vi "Print_Barcode.vi"(6 "RePrint":bool, 8 "error in (no error)":errorcluster, 9 "User Data":T1, 10 "RFID":string, 11 "Ref in":T2={"MS SQL Connection"=refnum, "UDL File"=path "", "Time"="", "DCODE"="", "WIP+1"=0, "MC No?"=0, "POKAYOKE?"=FALSE, "Expected Result"="", "Result [Status]"="", "Clock"=0.0, "RFID"="", "WIP Queue"=refnum, "TS Parameter"={"ProfitCenterCode"="", "LineCode"="", "WorkOrderNumber"="", "Model"="", "Model_with_Prefix"="", "VendorCode"="", "SetParameterDateCode"="", "PokaYoke"=0, "Target"=1, "Live_DateCode"="", "CustomerPartNumber"="", "Hand"="", "sBarcode"=FALSE, "FCA"=0, "Ent_Stamp"=timestamp(0 s since 1904-01-01), "STS_CD"=0.0}, "Data_Queue"=[], "RFID Serial No."=""} {"TS Parameter"."FCA" format="%01d"; "TS Parameter"."Target" min=1 max=100000; "TS Parameter"."PokaYoke" min=0 max=1}) -> (0 "error out":errorcluster, 1 "Serial No.":i32, 2 "Barcode":string, 3 "Ref Out":T2={"MS SQL Connection"=refnum, "UDL File"=path "", "Time"="", "DCODE"="", "WIP+1"=0, "MC No?"=0, "POKAYOKE?"=FALSE, "Expected Result"="", "Result [Status]"="", "Clock"=0.0, "RFID"="", "WIP Queue"=refnum, "TS Parameter"={"ProfitCenterCode"="", "LineCode"="", "WorkOrderNumber"="", "Model"="", "Model_with_Prefix"="", "VendorCode"="", "SetParameterDateCode"="", "PokaYoke"=0, "Target"=1, "Live_DateCode"="", "CustomerPartNumber"="", "Hand"="", "sBarcode"=FALSE, "FCA"=0, "Ent_Stamp"=timestamp(0 s since 1904-01-01), "STS_CD"=0.0}, "Data_Queue"=[], "RFID Serial No."=""} {"TS Parameter"."FCA" format="%01d"; "TS Parameter"."Target" min=1 max=100000; "TS Parameter"."PokaYoke" min=0 max=1}, 4 "Last Printed BC Mirror":string, 5 "Print Time":string, 7 "resulting string":string)   [LabVIEW 2020]
uses:
  Controls/TD SQL.ctl
  <vilib>/addons/database/Connection.llb/Conn ObjectReference.ctl
  Controls/WIP_State.ctl
  Controls/TS_Parameter.ctl
  Controls/user_log.ctl
  <vilib>/addons/database/Connection.llb/Conn Execute.vi
  <vilib>/addons/database/Recordset.llb/Rec Fetch Recordset Data (R).vi
  <vilib>/addons/database/Recordset.llb/Rec Destroy - Connection.vi
  <vilib>/addons/database/_DB Variant To Data/Database Variant To Data.xnode
  <vilib>/addons/database/NI_Database_API.lvlib
panel:
  out "match substring":string
  out "Pass Date":timestamp
  out "element":string
  out "Total Seconds 2":i32
  out "substring":string
  out "text 2":string
  out "Total Seconds":i32
  out "text":string
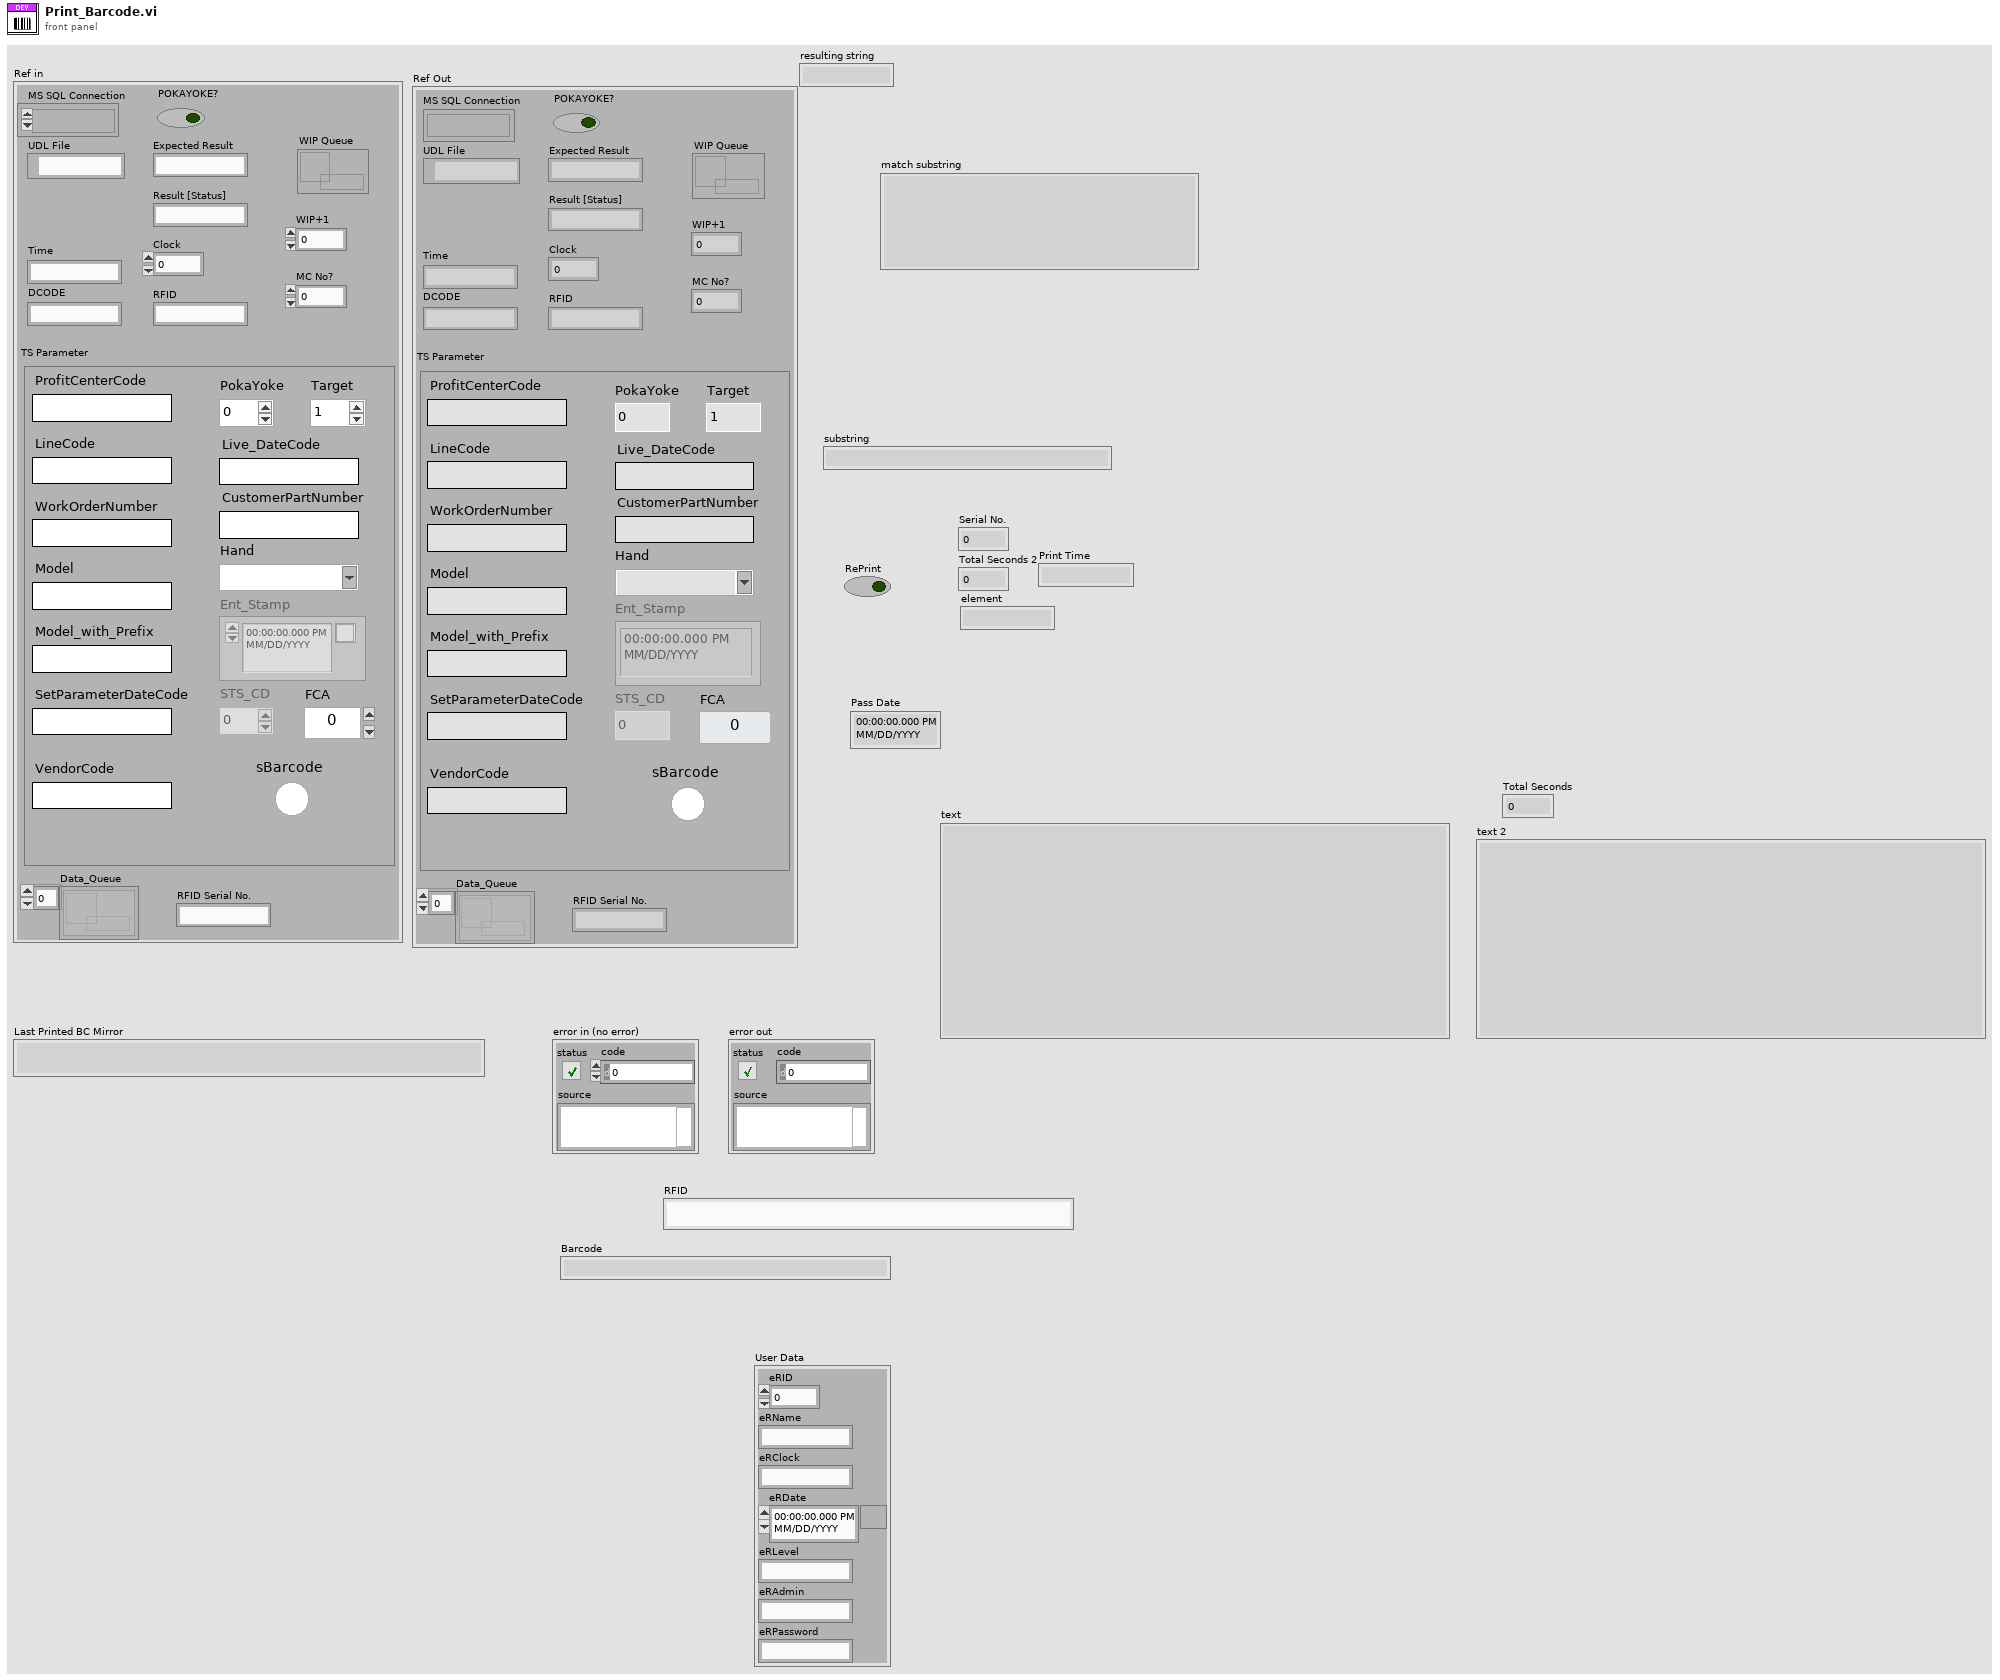
[diagram p1: front panel]
types:
  T1 = typedef "user_log.ctl" = cluster{"eRID":u16, "eRName":string, "eRClock":string, "eRDate":timestamp, "eRLevel":string, "eRAdmin":string, "eRPassword":string}
  T2 = typedef "TD SQL.ctl" = cluster{"MS SQL Connection":T3, "UDL File":path, "Time":string, "DCODE":string, "WIP+1":i64, "MC No?":i32, "POKAYOKE?":bool, "Expected Result":string, "Result [Status]":string, "Clock":dbl, "RFID":string, "WIP Queue":refnum<queue>, "TS Parameter":T4, "Data_Queue":refnum<queue>[], "RFID Serial No.":string}
  T3 = typedef "NI_Database_API.lvlib/Conn ObjectReference.ctl" = refnum<k1>
  T4 = typedef "TS_Parameter.ctl" = cluster{"ProfitCenterCode":string, "LineCode":string, "WorkOrderNumber":string, "Model":string, "Model_with_Prefix":string, "VendorCode":string, "SetParameterDateCode":string, "PokaYoke":i32, "Target":i32, "Live_DateCode":string, "CustomerPartNumber":string, "Hand":string, "sBarcode":bool, "FCA":i32, "Ent_Stamp":timestamp, "STS_CD":dbl}
  T5 = cluster{"CUSTOMER PART NUMBER":string, "Version Number":string, "VENDOR CODE":string, "BI PART NUMBER":string, "SCAN TYPE":enum16{"AUTO", "MANUAL"}, "BARCODE TYPE":enum16{"X451", "MSIL-YNC10 Trial1"}, "CELL NUMBER":string}
  T6 = enum16{"open", "replace", "create", "open or create", "replace or create", "replace or create with confirmation"}
  T7 = typedef "NI_Database_API.lvlib/Rec ObjectReference.ctl" = refnum<k1>
  T8 = cluster{"Data Path":path, "Calibration Path":path, "Settings Path":path, "Script Path":path, "DAQ Support":path, "Reporting Desktop":path, "Help":path}
  T9 = typedef "LVDateTimeRec.ctl" = cluster{"fractional second":dbl, "second":i32, "minute":i32, "hour":i32, "day of month":i32, "month":i32, "year":i32, "day of week":i32, "day of year":i32, "DST":i32}
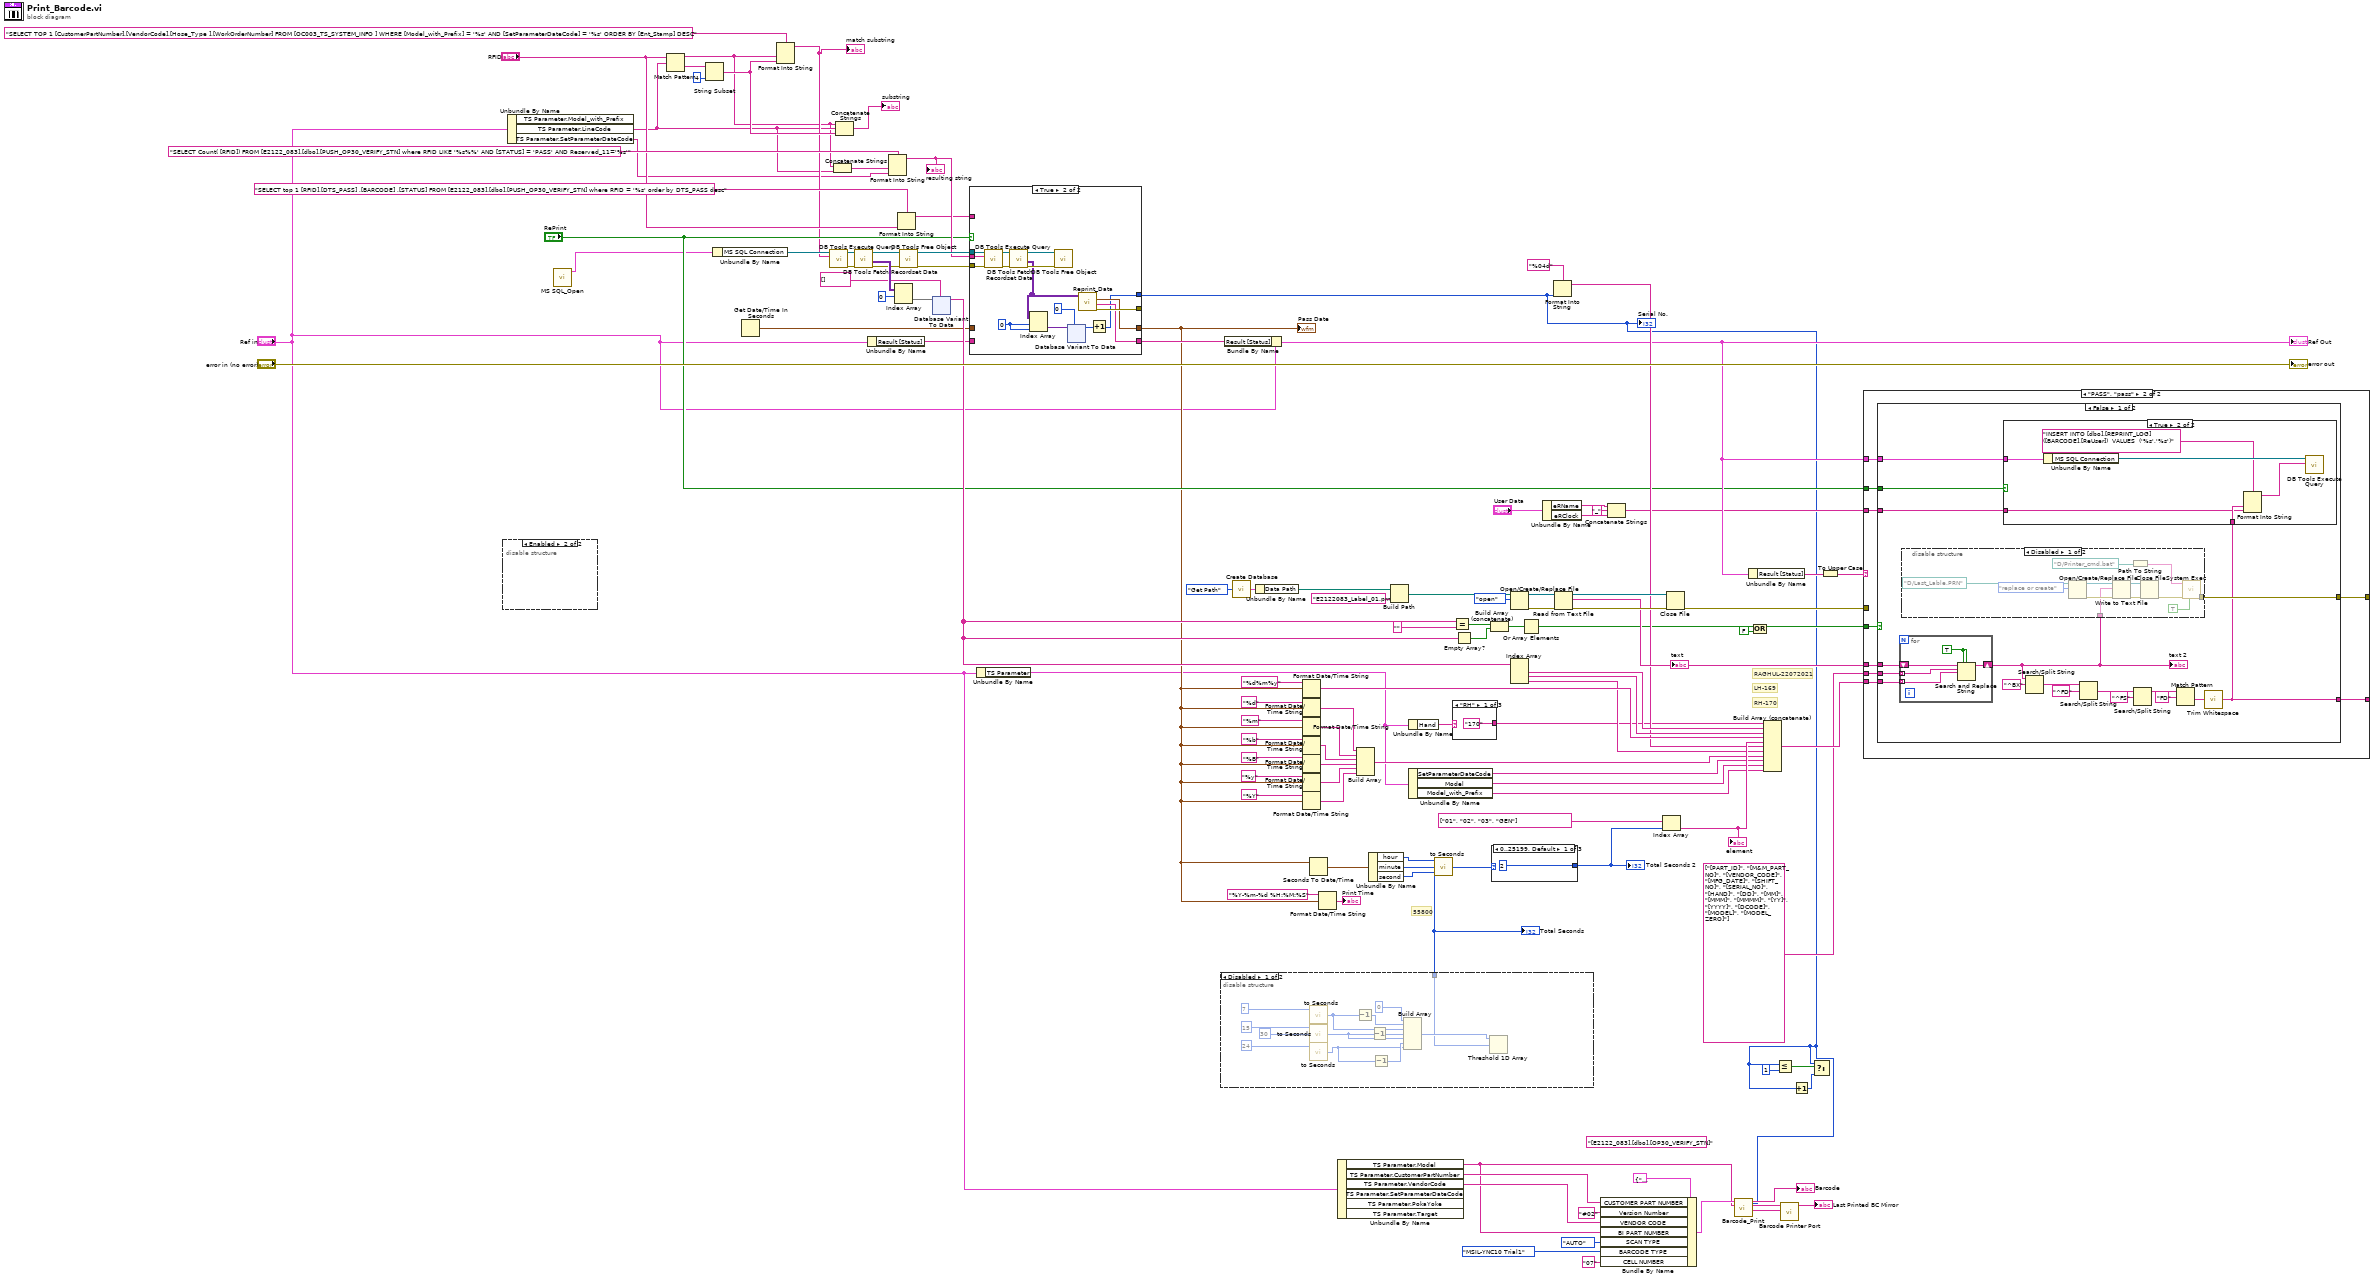
[diagram p0: block diagram]
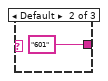
[diagram p2: hidden frame]
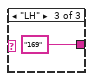
[diagram p3: hidden frame]
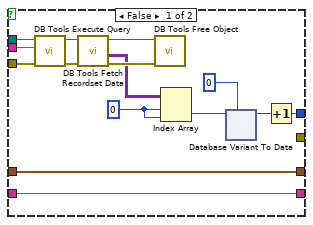
[diagram p5: hidden frame]
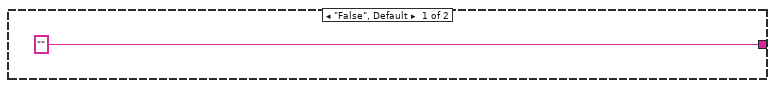
[diagram p6: hidden frame]
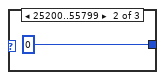
[diagram p11: hidden frame]
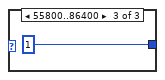
[diagram p12: hidden frame]
diagram:
  (unwired) "[E2122_083].[dbo].[OP30_VERIFY_STN]" ("table")
  # "RAGHUL-22072021"
  # "RH-170"
  # "LH-169"
  # "55800"
  n1 = disable-structure shown="Enabled" {
    frame Disabled {
    }
    frame Enabled {
    }
  }
  n2 = Unbundle By Name("Ref in") -> ("TS Parameter.LineCode"=w5:string, "TS Parameter.SetParameterDateCode"=w3:string)  [unwired: 1 out]
  n3 = call "MS SQL_Open.vi"() -> ("Ref Out"=w22:T2)  [unwired: 9 in, 2 out]
  n4 = Match Pattern(string="RFID", regular expression=w5) -> (before substring=w2:string, after substring=w76:string)  [unwired: 1 in, 2 out]
  n5 = String Subset(string=w76, length (rest)=4 ("length (rest)")) -> (substring=w59:string)  [unwired: 1 in]
  n6 = Unbundle By Name(w22) -> ("MS SQL Connection"=w68:T3)
  n7 = Get Date/Time In Seconds() -> (seconds since 1Jan1904=w35:timestamp)
  n8 = Format Into String(format string="SELECT TOP 1 [CustomerPartNumber],[VendorCode],[Hose_Type ],[WorkOrderNumber] FROM [OC003_TS_SYSTEM_INFO ] WHERE [Model_with_Prefix] = '%s' AND [SetParameterDateCode] = '%s' ORDER BY [Ent_Stamp] DESC" ("condition"), w2, w59) -> (resulting string=w23:string)  [unwired: 2 in, 1 out]
  "match substring" <- w23
  n9 = call-poly <vilib>:"DB Tools Execute Query.vi"("SQL query"=w23, "connection reference"=w68) -> ("error out"=w72:errorcluster, "recordset reference"=w73:T7)  [unwired: 6 in]
  n10 = Concatenate Strings(w2, w5) -> (w4:string)
  n11 = Concatenate Strings(w2, w5, w59) -> (→"substring":string)
  n12 = call-poly <vilib>:"DB Tools Fetch Recordset Data.vi"("error in (no error)"=w72, "recordset reference"=w73) -> ("error out"=w62:errorcluster, "recordset data"=w71:variant[][], "recordset reference out"=w63:T7)  [unwired: 3 in]
  n13 = Unbundle By Name("Ref in") -> ("Result [Status]"=w44:string)
  n14 = Format Into String(format string="SELECT Count( [RFID]) FROM [E2122_083].[dbo].[PUSH_OP30_VERIFY_STN] where RFID LIKE '%s%%' AND [STATUS] = 'PASS' AND Reserved_11='%s'" ("condition"), w4, w3) -> (resulting string=w56:string)  [unwired: 2 in, 1 out]
  "resulting string" <- w56
  n15 = Index Array(array=w71, index (row)=0) -> (element=w70:variant[])  [unwired: 1 in]
  n16 = Format Into String(format string="SELECT top 1 [RFID],[DTS_PASS] ,[BARCODE] ,[STATUS] FROM [E2122_083].[dbo].[PUSH_OP30_VERIFY_STN] where RFID = '%s' order by DTS_PASS desc" ("condition"), "RFID") -> (resulting string=w45:string)  [unwired: 2 in, 1 out]
  n17 = call-poly <vilib>:"DB Tools Free Object.vi"("error in (no error)"=w62, "recordset reference"=w63) -> ("error out"=w60:errorcluster, "connection reference"=w61:T3)  [unwired: 8 in]
  n18 = xnode "Database Variant To Data"("database variant"=w70, "type"=string[] [] ("columns")) -> ("data"=w55:string[])  [unwired: 1 in, 1 out]
  n19 = case shown="True" "RePrint" {
    tunnel: w61 -> [w131 w179]
    tunnel: w60 -> [w130 w178]
    tunnel: w56 -> [w120 w170]
    tunnel: [w119 w164] -> w1
    tunnel: w45 -> [_ _]
    tunnel: [_ w173] -> _
    tunnel: w35 -> [w118 _]
    tunnel: [w118 w172] -> w32
    tunnel: w44 -> [w117 _]
    tunnel: [w117 w171] -> w43
    frame False {
      w123 = 0 ("index (row)")
      n20 = call-poly <vilib>:"DB Tools Execute Query.vi"("error in (no error)"=w130, "SQL query"=w120, "connection reference"=w131) -> ("error out"=w127:errorcluster, "recordset reference"=w128:T7)  [unwired: 5 in]
      n21 = call-poly <vilib>:"DB Tools Fetch Recordset Data.vi"("error in (no error)"=w127, "recordset reference"=w128) -> ("error out"=w126:errorcluster, "recordset data"=w124:variant[][], "recordset reference out"=w129:T7)  [unwired: 3 in]
      n22 = call-poly <vilib>:"DB Tools Free Object.vi"("error in (no error)"=w126, "recordset reference"=w129) -> ()  [unwired: 8 in, 2 out]
      n23 = Index Array(array=w124, index (row)=w123, index (col)=w123) -> (element=w125:variant)
      n24 = xnode "Database Variant To Data"("database variant"=w125, "type"=0 ("index (row)")) -> ("data"=w121:i32)  [unwired: 1 in, 1 out]
      n25 = Increment(x=w121) -> (x+1=w119:i32)
    }
    frame True {
      w166 = 0 ("index (row)")
      n26 = call-poly <vilib>:"DB Tools Execute Query.vi"("error in (no error)"=w178, "SQL query"=w170, "connection reference"=w179) -> ("error out"=w175:errorcluster, "recordset reference"=w176:T7)  [unwired: 5 in]
      n27 = call-poly <vilib>:"DB Tools Fetch Recordset Data.vi"("error in (no error)"=w175, "recordset reference"=w176) -> ("error out"=w174:errorcluster, "recordset data"=w165:variant[][], "recordset reference out"=w177:T7)  [unwired: 3 in]
      n28 = Index Array(array=w165, index (row)=w166, index (col)=w166) -> (element=w169:variant)
      n29 = call-poly <vilib>:"DB Tools Free Object.vi"("error in (no error)"=w174, "recordset reference"=w177) -> ()  [unwired: 8 in, 2 out]
      n30 = xnode "Database Variant To Data"("database variant"=w169, "type"=0 ("index (row)")) -> ("data"=w168:i32)  [unwired: 1 in, 1 out]
      n31 = call "Reprint_Data.vi"("recordset data"=w165) -> ("error out"=w173:errorcluster, "Status"=w171:string, "Pass Date"=w172:timestamp)  [unwired: 5 in, 3 out]
      n32 = Increment(x=w168) -> (x+1=w164:i32)
    }
  }
  "Serial No." <- w1
  "Pass Date" <- w32
  n33 = Unbundle By Name("Ref in") -> ("TS Parameter"=w26:T4)
  n34 = Bundle By Name(cluster="Ref in", "Result [Status]"=w43) -> (w42:T2)
  "Ref Out" <- w42
  n35 = call <userlib>:"Create Database.vi"("Get/Create"=enum16{"Get Path", "Create Path"}."Get Path") -> ("Path Out"=w110:T8)  [unwired: 13 in, 1 out]
  n36 = Unbundle By Name(w110) -> ("Data Path"=w109:path)
  n37 = Format Date/Time String(time format string (%c)="%d%m%y", seconds (now)=w32) -> (date/time string=w104:string)  [unwired: 1 in]
  n38 = Format Date/Time String(time format string (%c)="%d", seconds (now)=w32) -> (date/time string=w94:string)  [unwired: 1 in]
  n39 = Format Date/Time String(time format string (%c)="%m", seconds (now)=w32) -> (date/time string=w93:string)  [unwired: 1 in]
  n40 = Format Date/Time String(time format string (%c)="%b", seconds (now)=w32) -> (date/time string=w92:string)  [unwired: 1 in]
  n41 = Format Date/Time String(time format string (%c)="%B", seconds (now)=w32) -> (date/time string=w91:string)  [unwired: 1 in]
  n42 = Format Date/Time String(time format string (%c)="%y", seconds (now)=w32) -> (date/time string=w90:string)  [unwired: 1 in]
  n43 = Format Date/Time String(time format string (%c)="%Y", seconds (now)=w32) -> (date/time string=w89:string)  [unwired: 1 in]
  n44 = Seconds To Date/Time(time stamp (now)=w32) -> (date time rec=w87:T9)  [unwired: 1 in]
  n45 = Format Date/Time String(time format string (%c)="%Y-%m-%d %H:%M:%S", seconds (now)=w32) -> (date/time string=→"Print Time":string)  [unwired: 1 in]
  n46 = Unbundle By Name("Ref in") -> ("TS Parameter.Model"=w16:string, "TS Parameter.CustomerPartNumber"=w18:string, "TS Parameter.VendorCode"=w17:string)  [unwired: 3 out]
  n47 = Build Array(w94, w93, w92, w91, w90, w89) -> (w88:string[])
  n48 = Unbundle By Name(w87) -> ("hour"=w86:i32, "minute"=w31:i32, "second"=w30:i32)
  n49 = Build Path(base path=w109, name or relative path="E2122083_Label_01.prn") -> (appended path=w107:path)
  n50 = Unbundle By Name(w26) -> ("Hand"=w25:string)
  n51 = Unbundle By Name(w26) -> ("SetParameterDateCode"=w29:string, "Model"=w28:string, "Model_with_Prefix"=w27:string)
  n52 = call "to Seconds.vi"("Minute"=w30, "Second"=w31, "Hour"=w86) -> ("Total Seconds"=w85:i32)
  "Total Seconds" <- w85
  n53 = disable-structure shown="Disabled" {
    disable-tunnel: w85 -> [w212 _]
    frame Disabled {
      n54 = call "to Seconds.vi"("Hour"=7 ("length (rest)")) -> ("Total Seconds"=w218:i32)  [unwired: 2 in]
      n55 = call "to Seconds.vi"("Second"=30 ("length (rest)"), "Hour"=15 ("length (rest)")) -> ("Total Seconds"=w216:i32)  [unwired: 1 in]
      n56 = call "to Seconds.vi"("Hour"=24 ("length (rest)")) -> ("Total Seconds"=w213:i32)  [unwired: 2 in]
      n57 = Decrement(x=w218) -> (x-1=w217:i32)
      n58 = Decrement(x=w216) -> (x-1=w215:i32)
      n59 = Decrement(x=w213) -> (x-1=w214:i32)
      n60 = Build Array(0 ("element"), w217, w218, w215, w216, w214, w213) -> (w220:i32[])
      n61 = Threshold 1D Array(2:w212, 3:w220) -> ()  [unwired: 1 in, 1 out]
    }
    frame Enabled {
    }
  }
  n62 = case shown="\"RH\"" w25 {
    tunnel: ["170" ("spreadsheet string") "601" ("spreadsheet string") "169" ("spreadsheet string")] -> w24
    frame "RH" {
    }
    frame Default {
    }
    frame "LH" {
    }
  }
  n63 = Equal?(x=w55, y="" ("element")) -> (x = y?=w53:bool[])
  n64 = Empty Array?(array=w55) -> (empty?=w51:bool)
  n65 = Build Array (concatenate)(w53, w51) -> (w52:bool[])
  n66 = case shown="0..25199, Default" w85 {
    tunnel: [2 ("Total Seconds") 0 ("Total Seconds") 1 ("Total Seconds")] -> w84
    frame 0..25199, Default {
    }
    frame 25200..55799 {
    }
    frame 55800..86400 {
    }
  }
  "Total Seconds 2" <- w84
  n67 = Open/Create/Replace File(file path (use dialog)=w107, operation (0:open)=T6."open") -> (refnum out=w114:refnum<file>, error out=w115:errorcluster)  [unwired: 4 in, 1 out]
  n68 = Index Array(array=w55) -> (element #1=w67:string, element #2=w66:string, element #3=w65:string)  [unwired: 3 in]
  n69 = Or Array Elements(Boolean array=w52) -> (logical OR=w50:bool)
  n70 = Unbundle By Name("User Data") -> ("eRName"=w39:string, "eRClock"=w38:string)
  n71 = Format Into String(format string="%04d", w1) -> (resulting string=w64:string)  [unwired: 2 in, 1 out]
  n72 = Read from Text File(file (use dialog)=w114, error in=w115) -> (refnum out=w113:refnum<file>, text=w81:string, error out=w112:errorcluster)  [unwired: 2 in, 1 out]
  "text" <- w81
  n73 = Bundle By Name(cluster=T5 {"CUSTOMER PART NUMBER"="106", "Version Number"="106", "VENDOR CODE"="106", "BI PART NUMBER"="106", "SCAN TYPE"=enum."AUTO", "BARCODE TYPE"=enum."X451", "CELL NUMBER"=""} ("Parameter"), "CUSTOMER PART NUMBER"=w18, "Version Number"="#02", "VENDOR CODE"=w17, "BI PART NUMBER"=w16, "SCAN TYPE"=enum16{"AUTO", "MANUAL"}."AUTO", "BARCODE TYPE"=enum16{"X451", "MSIL-YNC10 Trial1"}."MSIL-YNC10 Trial1", "CELL NUMBER"="07") -> (w19:T5)
  n74 = Concatenate Strings(w39, "_" ("string"), w38) -> (w36:string)
  n75 = Index Array(array=string[] ["01", "02", "03", "GEN"], index=w84) -> (element=w102:string)
  "element" <- w102
  n76 = Close File(refnum=w113, error in=w112) -> (error out=w80:errorcluster)  [unwired: 1 out]
  n77 = call "Barcode_Print"("Slno"=w1, "Ring Text.Text"=w16, "Parameter"=w19) -> ("Text Command for Printer"=w21:string, "Last Printed BC Mirror"=→"Last Printed BC Mirror":string, "Last Printed Barcode"=→"Barcode":string)  [unwired: 6 in]
  n78 = Unbundle By Name(w42) -> ("Result [Status]"=w79:string)
  n79 = Compound Arithmetic op=OR(w50, FALSE ("value")) -> (w49:bool)
  n80 = Build Array (concatenate)(w24, w67, w66, w104, w102, w64, w65, w88, w29, w28, w27) -> (w83:string[])
  n81 = Less Or Equal?(x=w1, y=1) -> (x <= y?=w7:bool)
  n82 = call "Barcode Printer Port.vi"("string to write"=w21) -> ()  [unwired: 10 in, 1 out]
  n83 = Increment(x=w1) -> (x+1=w6:i32)
  n84 = Select(t=w1, s=w7, f=w6) -> ()  [unwired: 1 out]
  n85 = To Upper Case(1:w79) -> (0:w78:string)
  n86 = case shown="\"PASS\", \"pass\"" w78 {
    tunnel: w83 -> [_ w240]
    tunnel: string[] ["[PART_ID]", "[M&M_PART_NO]", "[VENDOR_CODE]", "[MFG_DATE]", "[SHIFT_NO]", "[SERIAL_NO]", "[HAND]", "[DD]", "[MM]", "[MMM]", "[MMMM]", "[YY]", "[YYYY]", "[DCODE]", "[MODEL]", "[MODEL_ZERO]"] ("array") -> [_ w239]
    tunnel: w81 -> [_ w238]
    tunnel: w80 -> [_ _]
    tunnel: ["" ("trimmed string") w237] -> _
    tunnel: [_ w236] -> _
    tunnel: w49 -> [_ w235]
    tunnel: w42 -> [_ w234]
    tunnel: "RePrint" -> [_ w233]
    tunnel: w36 -> [_ w232]
    frame "False", Default {
    }
    frame "PASS", "pass" {
      n87 = case shown="False" w235 {
        tunnel: w240 -> [w257 _]
        tunnel: w239 -> [w256 _]
        tunnel: w238 -> [w255 _]
        tunnel: [w244 _] -> w237
        tunnel: [w245 _] -> w236
        tunnel: w234 -> [w243 _]
        tunnel: w233 -> [w242 _]
        tunnel: w232 -> [w241 _]
        frame False {
          n88 = for {
            shift-right: [w277] -> w251
            shift-left: w255 -> [w280]
            tunnel: w257 -> [w279] mode=indexing
            tunnel: w256 -> [w278] mode=indexing
            w276 = TRUE ("replace all? (F)")
            n89 = Search and Replace String(replace all?=w276, case sensitive?=w276, input string=w280, search string=w278, replace string=w279) -> (result string=w277:string)  [unwired: 3 in, 3 out]
          }
          "text 2" <- w251
          n90 = disable-structure shown="Disabled" {
            disable-tunnel: w251 -> [w260 _]
            disable-tunnel: [w259 _] -> w245
            frame Disabled {
              n91 = Open/Create/Replace File(file path (use dialog)=path "D:/Last_Lable.PRN" ("appended path"), operation (0:open)=T6."replace or create") -> (refnum out=w266:refnum<file>, error out=w265:errorcluster)  [unwired: 4 in, 1 out]
              n92 = Write to Text File(file (use dialog)=w266, text=w260, error in=w265) -> (refnum out=w267:refnum<file>, error out=w268:errorcluster)  [unwired: 1 in, 1 out]
              n93 = Path To String(path=path "D:/Printer_cmd.bat" ("appended path")) -> (string=w261:string)
              n94 = Close File(refnum=w267, error in=w268) -> (error out=w263:errorcluster)  [unwired: 1 out]
              n95 = call <vilib>:"System Exec.vi"("run minimized? (F)"=TRUE, "error in (no error)"=w263, "command line"=w261) -> ("error out"=w259:errorcluster)  [unwired: 5 in, 3 out]
            }
            frame Enabled {
            }
          }
          n96 = Search/Split String(string=w251, search string/char (-)="^BX" ("regular expression")) -> (match + rest of string=w254:string)  [unwired: 1 in, 2 out]
          n97 = Search/Split String(string=w254, search string/char (-)="^FD" ("regular expression")) -> (match + rest of string=w253:string)  [unwired: 1 in, 2 out]
          n98 = Search/Split String(string=w253, search string/char (-)="^FS" ("regular expression")) -> (substring before match=w249:string)  [unwired: 1 in, 2 out]
          n99 = Match Pattern(string=w249, regular expression="FD") -> (after substring=w247:string)  [unwired: 1 in, 3 out]
          n100 = call <vilib>:"Trim Whitespace.vi"("string"=w247) -> ("trimmed string"=w244:string)  [unwired: 1 in]
          n101 = case shown="True" w242 {
            tunnel: w244 -> [_ w272]
            tunnel: w243 -> [_ w271]
            tunnel: w241 -> [_ w270]
            frame False {
            }
            frame True {
              n102 = Unbundle By Name(w271) -> ("MS SQL Connection"=w275:T3)
              n103 = Format Into String(format string="INSERT INTO [dbo].[REPRINT_LOG] ([BARCODE],[ReUser])  VALUES  ('%s','%s')" ("SQL query"), w272, w270) -> (resulting string=w273:string)  [unwired: 2 in, 1 out]
              n104 = call-poly <vilib>:"DB Tools Execute Query.vi"("SQL query"=w273, "connection reference"=w275) -> ()  [unwired: 6 in, 2 out]
            }
          }
        }
        frame True {
        }
      }
    }
  }
  "error out" <- "error in (no error)"
